vi "Close Door.vi"(8 "error in (no error)":errorcluster, 11 "Doors Closing in":refnum<class "Doors Closing.lvclass">) -> (0 "error out":errorcluster, 3 "Doors Closing out":refnum<class "Doors Closing.lvclass">)   [LabVIEW 2020, in "Door Controller.lvlib" / "Doors Closing.lvclass"]
uses:
  Doors Closing.lvclass
  Door Controller/Door Controller.lvclass
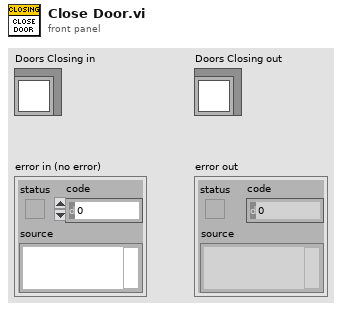
[diagram p1: front panel]
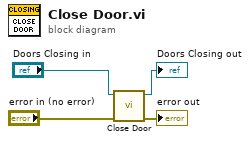
[diagram p0: block diagram]
diagram:
  n1 = call-parent "Close Door.vi"("error in (no error)"="error in (no error)", "Door Controller in"="Doors Closing in") -> ("error out"=→"error out":errorcluster, "Door Controller out"=→"Doors Closing out":refnum<class "Doors Closing.lvclass">)  [unwired: 8 in]
